vi "NI Get Window RefNum.vi"(8 "error in (no error)":errorcluster, 11 "window name (\"\")":string) -> (0 "error out":errorcluster, 3 "window refnum (NaWR)":refnum<k1>)   [LabVIEW 2018]
doc: "This VI will use the FindWindow API function to retrieve a window refnum for the window identified by window name. 'window name' is the text appearing in the title bar of a window. If the window cannot be found, the window refnum out will be 'Not a Window Refnum', and an error will occur."
uses:
  user32.dll
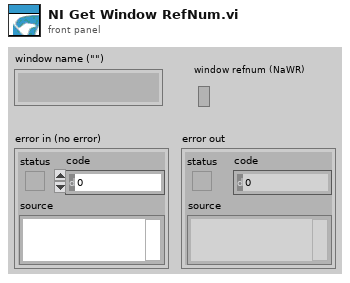
[diagram p1: front panel]
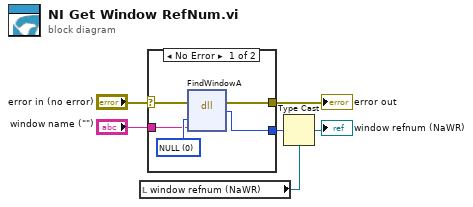
[diagram p0: block diagram]
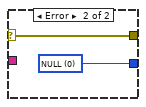
[diagram p2: hidden frame]
diagram:
  n1 = local read "window refnum (NaWR)"() -> (w4:refnum<k1>)
  n2 = case shown="No Error" "error in (no error)" {
    selector: "error in (no error)" -> [w8 w12]
    tunnel: [w7 w12] -> w1
    tunnel: [w11 w13] -> w6
    tunnel: "window name (\"\")" -> [w9 _]
    frame No Error {
      w10 = 0 items=["NULL"]
      n3 = dll-call lib="user32.dll" fn="FindWindowA" label="FindWindow"(error in=w8, "lpszClassName"=w10, "lpszWindowName"=w9) -> (error out=w7:errorcluster, "hWnd"=w11:u32)  [unwired: 4 in, 1 out]
    }
    frame Error {
      w13 = u16 0 items=["NULL"]
    }
  }
  "error out" <- w1
  n4 = Type Cast(type=w4, x=w6) -> (*(type *) &x=→"window refnum (NaWR)":refnum<k1>)
